vi "bookmarker.vi"() -> ()   [LabVIEW 2012]
doc: "This very simple code can be used to allow the scrollbar to be made sepirate from an array"
panel:
  in  "VISA resource name":refnum<visa-resource-name>="COM17"
  in  "OK Button":bool
  in  "Multicolumn Listbox":i32(listbox)
  in  "stop":bool
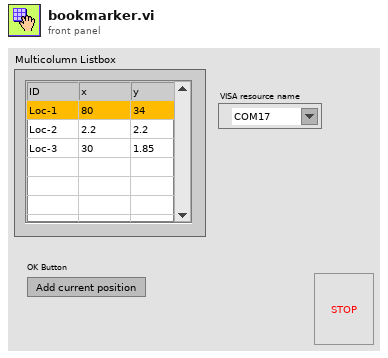
[diagram p1: front panel]
types:
  T1 = typedef "LVPoint32TypeDef.ctl" = cluster{"Horizontal":i32, "Vertical":i32}
  T2 = typedef "LVRowAndColumnTypeDef.ctl" = cluster{"Row":i32, "Column":i32}
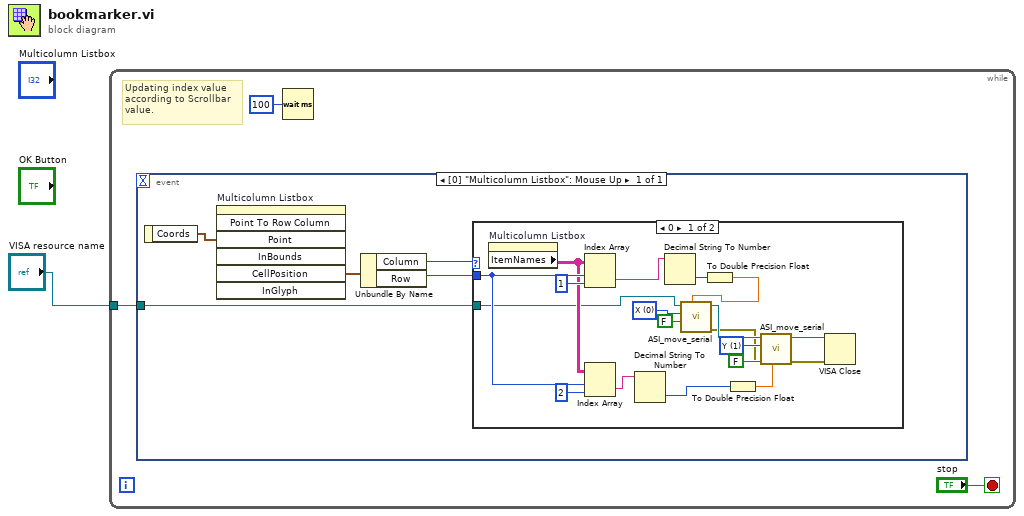
[diagram p0: block diagram]
diagram:
  n1 = while {
    tunnel: "VISA resource name" -> [w2]
    stop <- "stop" stop-if-true
    # "Updating index value according to Scrollbar value."
    n2 = event shown="[0] \"Multicolumn Listbox\": Mouse Up" {
      selector: _ -> [_]
      dyn-events: _ -> [_]
      timeout: _ -> [_]
      tunnel: w2 -> [w5]
      event "Multicolumn Listbox": Mouse Up {
        n3 = event-data() -> ("Coords"=w9:T1)  [unwired: 1 in]
        n4 = invoke on="Multicolumn Listbox" class="MCListbox (strict)" method="Point To Row Column"("Point"=w9) -> ("CellPosition"=w8:T2)  [unwired: 6 in, 6 out]
        n5 = Unbundle By Name(w8) -> ("Column"=w7:i32, "Row"=w6:i32)
        n6 = case shown="0" w7 {
          tunnel: w6 -> [w26 _]
          tunnel: w5 -> [w10 _]
          frame 0 {
            w20 = u16 1 items=["X", "Y", "Z"] ("Axis")
            w28 = u16 0 items=["X", "Y", "Z"] ("Axis")
            n7 = property on="Multicolumn Listbox" class="MCListbox (strict)"() -> ("ItemNames"=w24:string[][])  [unwired: 2 in, 2 out]
            n8 = Index Array(array=w24, index (row)=w26, index (col)=1 ("disabled index (col)")) -> (element=w23:string)
            n9 = Index Array(array=w24, index (row)=w26, index (col)=2 ("disabled index (col)")) -> (element=w18:string)
            n10 = Decimal String To Number(string=w18) -> (number=w13:i32)  [unwired: 2 in, 1 out]
            n11 = Decimal String To Number(string=w23) -> (number=w16:i32)  [unwired: 2 in, 1 out]
            n12 = To Double Precision Float(number=w16) -> (double precision float=w15:dbl)
            n13 = call "ASI_move_serial.vi"("Position/distance (um)"=w15, "Relative?"=FALSE, "Axis"=w28, "VISA resource name"=w10) -> ("error out"=w17:errorcluster, "VISA resource name out"=w21:refnum<visa-resource-name>)  [unwired: 3 in]
            n14 = To Double Precision Float(number=w13) -> (double precision float=w14:dbl)
            n15 = call "ASI_move_serial.vi"("Position/distance (um)"=w14, "error in"=w17, "Relative?"=FALSE, "Axis"=w20, "VISA resource name"=w21) -> ("error out"=w11:errorcluster, "VISA resource name out"=w12:refnum<visa-resource-name>)  [unwired: 2 in]
            n16 = VISA Close(VISA resource name=w12, error in (no error)=w11) -> ()  [unwired: 1 out]
          }
          frame Default {
          }
        }
      }
    }
    n17 = Wait (ms)(milliseconds to wait=u32 100) -> ()  [unwired: 1 out]
  }
